vi "Write Process Name.vi"(0 "Process Out":refnum<class "Process.lvclass">, 5 "Process Name":string, 11 "Error In":errorcluster) -> (4 "Process Out":refnum<class "Process.lvclass">, 15 "Error Out":errorcluster)   [LabVIEW 2023, in "Process.lvclass"]
uses:
  Process.lvclass
  Process.lvclass/Process.ctl
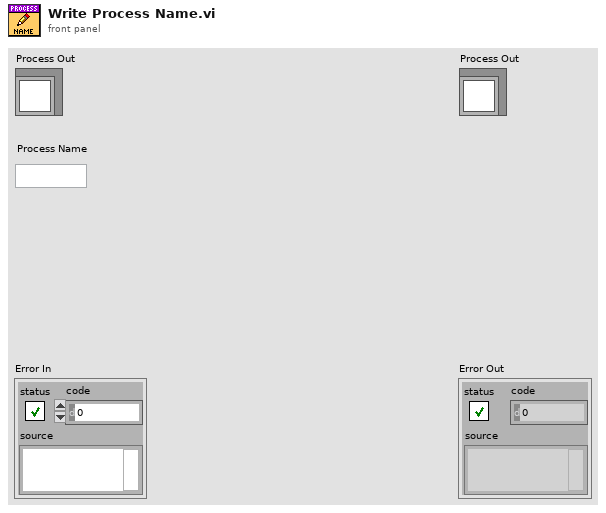
[diagram p1: front panel]
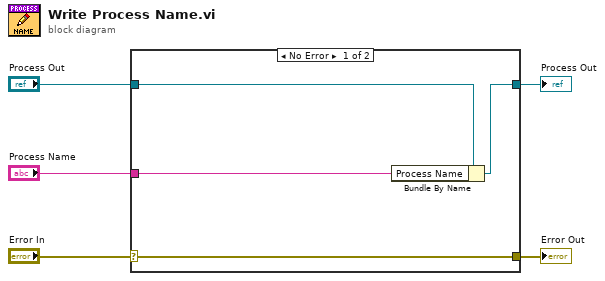
[diagram p0: block diagram]
diagram:
  n1 = case shown="No Error" "Error In" {
    selector: "Error In" -> [w9 w10]
    tunnel: [w9 w10] -> w4
    tunnel: [w7 w11] -> w2
    tunnel: "Process Out" -> [w8 w11]
    tunnel: "Process Name" -> [w6 _]
    frame No Error {
      n2 = Bundle By Name(cluster=w8, "Process Name"=w6) -> (w7:refnum<class "Process.lvclass">)
    }
    frame Error {
    }
  }
  "Error Out" <- w4
  "Process Out" <- w2
